vi "DAQ Engine Stop Post Sub Steps.vi"(10 "DAQ Engine":string(combo), 11 "Sequence Context In":refnum<k7>) -> (0 "error out":errorcluster, 3 "Report Text":string)   [LabVIEW 2023, in "LTT_TeststandSteptypes.lvlib"]
uses:
  LTT_TeststandSteptypes.lvlib
  DAQ Engine.vi
  <vilib>/addons/TestStand/_TSUtility.llb/TestStand - Get Property Value (Number {Signed 16-bit Integer}).vi
  HardwareAbstractionLayer_LVOOP/Teststand/Teststand Engine Driver/Control/Teststand Status Control.ctl
  HardwareAbstractionLayer_LVOOP/Teststand/Teststand.lvclass
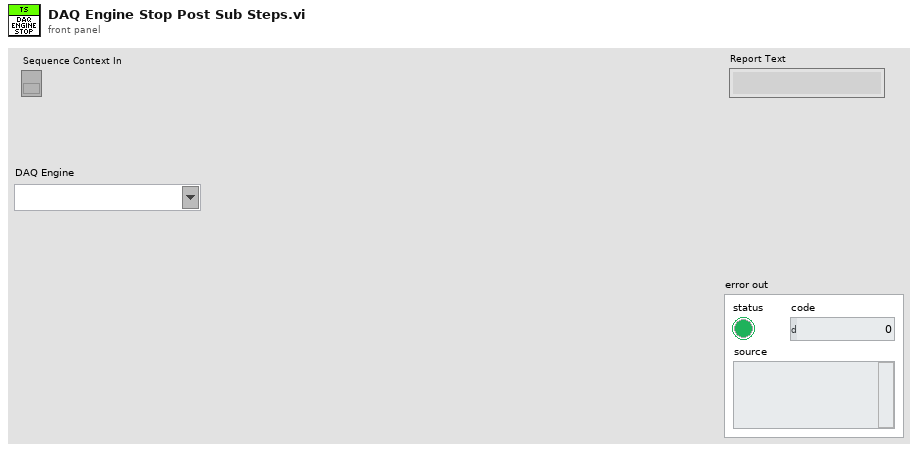
[diagram p1: front panel]
types:
  T1 = typedef "HardwareAbstractionLayer_LVOOP.lvlib/Teststand.lvclass/Teststand Status Control.ctl" = cluster{"Terminating or Aborting":bool, "Stop":bool, "Socket Count":i16, "Selected Sockets":i16[]}
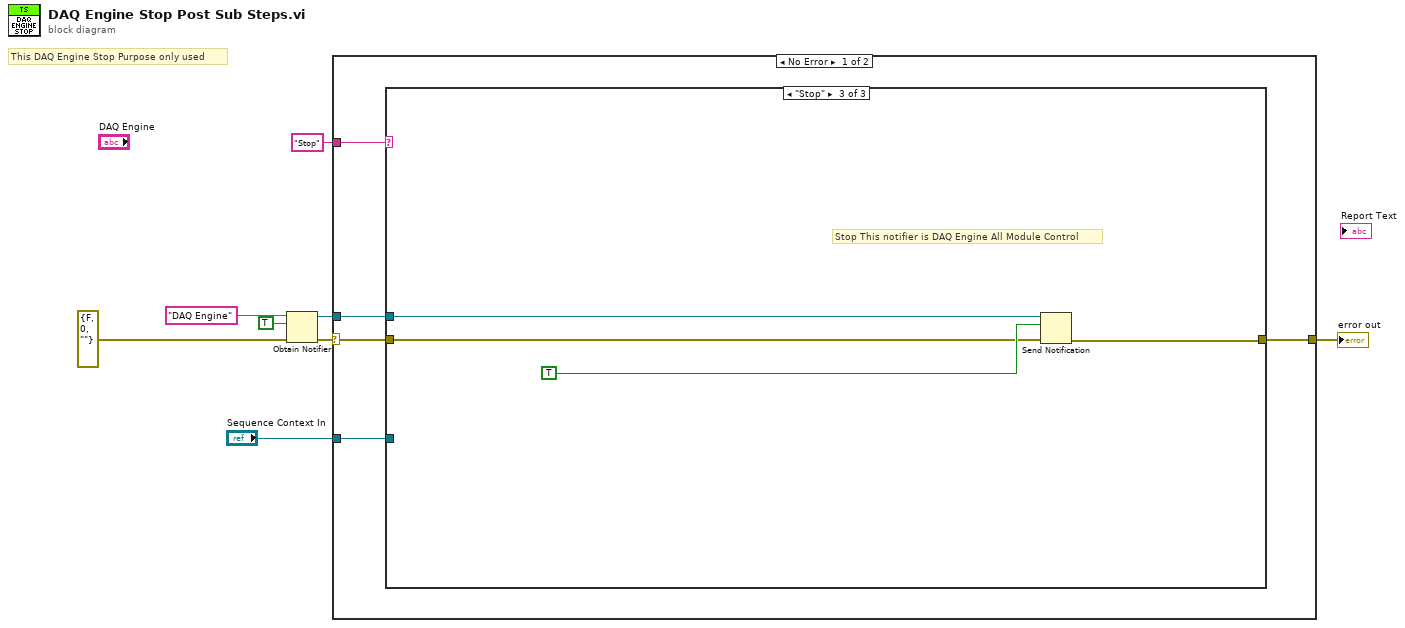
[diagram p0: block diagram]
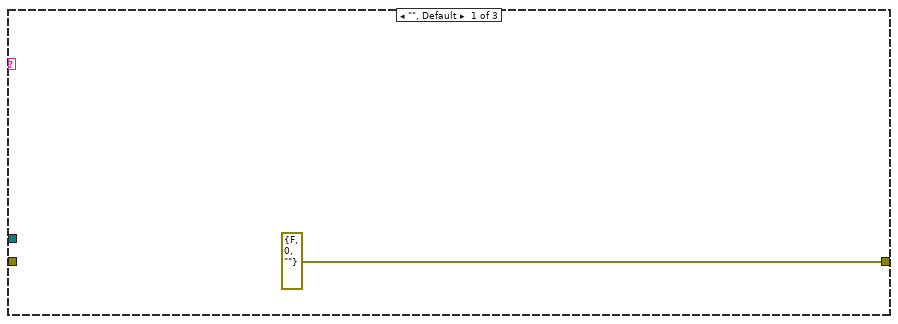
[diagram p2: hidden frame]
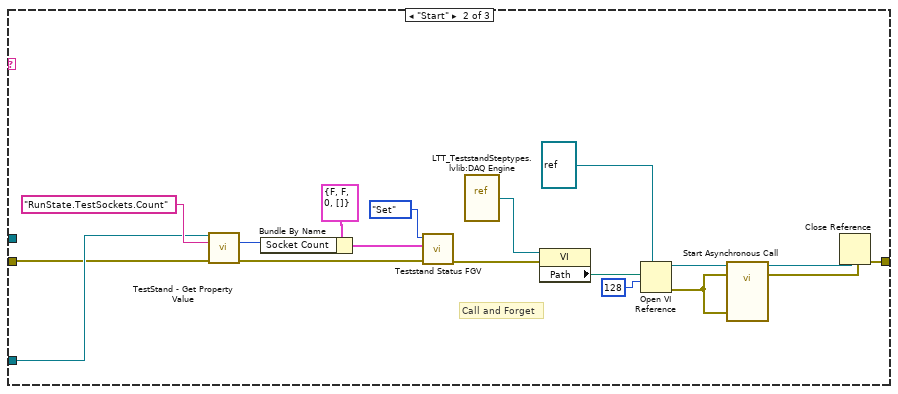
[diagram p3: hidden frame]
diagram:
  # "This DAQ Engine Stop Purpose only used"
  n1 = Obtain Notifier(name (unnamed)="DAQ Engine", notification data type=TRUE, error in (no error)=errorcluster {"status"=FALSE, "code"=0, "source"=""} ("error in")) -> (notifier out=w3:refnum<notifier>, error out=w2:errorcluster)  [unwired: 1 in, 1 out]
  n2 = case shown="No Error" w2 {
    selector: w2 -> [w9 w37]
    tunnel: "Stop" ("DAQ Engine") -> [w13 _]
    tunnel: [w12 w37] -> w8
    tunnel: "Sequence Context In" -> [w11 _]
    tunnel: w3 -> [w10 _]
    frame No Error {
      n3 = case shown="\"Stop\"" w13 {
        tunnel: [errorcluster {"status"=FALSE, "code"=0, "source"=""} ("error out") w20 w34] -> w12
        tunnel: w11 -> [_ w24 _]
        tunnel: w10 -> [_ _ w36]
        tunnel: w9 -> [_ w18 w33]
        frame "", Default {
        }
        frame "Start" {
          # "Call and Forget"
          n4 = call-poly <vilib>:"TestStand - Get Property Value.vi"("Sequence Context In"=w24, "Lookup String"="RunState.TestSockets.Count", "error in (no error)"=w18) -> ("Value"=w16:i16, "error out"=w19:errorcluster)  [unwired: 10 in, 1 out]
          n5 = Bundle By Name(cluster=T1 {"Terminating or Aborting"=FALSE, "Stop"=FALSE, "Socket Count"=0, "Selected Sockets"=[]} ("Teststand Status"), "Socket Count"=w16) -> (w15:T1)
          n6 = call "Teststand Status FGV.vi"("error in"=w19, "Teststand Status"=w15, "Option"=enum16{"Set", "Get"}."Set") -> ("error out"=w21:errorcluster)  [unwired: 7 in, 1 out]
          n7 = vi-ref "LTT_TeststandSteptypes.lvlib:DAQ Engine.vi"() -> (w32:refnum<vi>)
          n8 = property class="VI"(reference=w32, error in=w21) -> ("Path"=w31:path)  [unwired: 2 out]
          n9 = Open VI Reference(type specifier VI Refnum (for type only)=refnum<vi> refnum, vi path=w31, options=128) -> (vi reference=w29:refnum<vi>, error out=w23:errorcluster)  [unwired: 3 in]
          n10 = call-by-ref "Start Asynchronous Call"(reference=w29, error in=w23, "error in"=w23) -> (reference out=w26:refnum<vi>, error out=w27:errorcluster)  [unwired: 10 in, 1 out]
          n11 = Close Reference(reference=w26, error in (no error)=w27) -> (error out=w20:errorcluster)
        }
        frame "Stop" {
          # "Stop This notifier is DAQ Engine All Module Control"
          n12 = Send Notification(notification=TRUE, notifier=w36, error in (no error)=w33) -> (error out=w34:errorcluster)  [unwired: 1 out]
        }
      }
    }
    frame Error {
    }
  }
  "error out" <- w8
